vi "1-1.vi"() -> ()   [LabVIEW 2012]
doc: "© Copyright M. Ferrari 2000"
panel:
  out "LED":bool caption="Modificare le dimensioni e il colore del LED evidenziare il testo booleano. Provare, tramite l'opzione Show... a far apparire e scomparire tali informazioni"
  in  "?":dbl(knob)=12.0 min=12.0 max=35.0 scale=0.0..10.0 scale format="%.1f"
  out "Graph":dbl(graph) caption="Modificare i parametri del grafico: scale e colori"
  in  "?":bool
  in  "?":bool
  in  "Etichetta":dbl format="%.2f"
  in  "?":bool
  in  "?":bool
  in  "?":bool
  in  "?":bool
  in  "?":bool
  in  "?":bool
  # "ESERCIZIO 1-1"
  # "Assegnare un' etichetta\ne cancellare questa scritta"
  # "Riposizionare unitariamente\ni 4 interruttori"
  # "Creare un'etichetta libera e duplicarla,\nmodificando i font della copia"
  # "Modificare i limiti e provare a ruotare la manopola"
  # "Questa è un'etichetta libera, fare in modo\nche rimanga il testo senza cornice"
  # "Allineare orizzontalmente i 4 pulsanti ed equispaziarli."
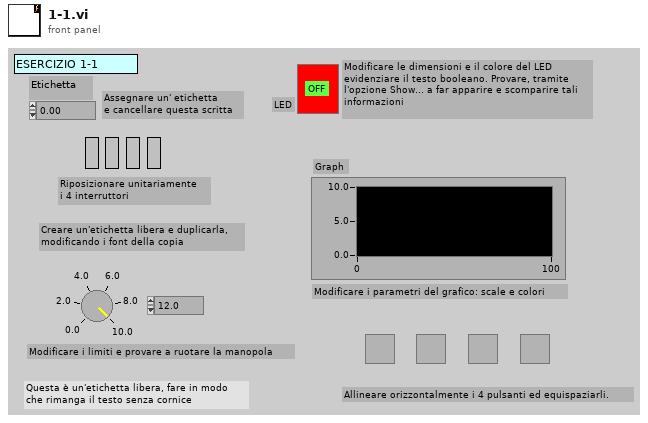
[diagram p1: front panel]
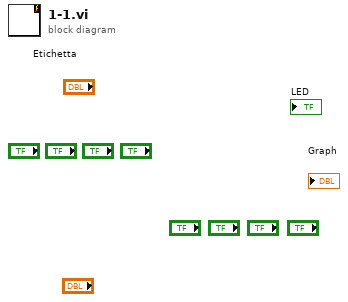
[diagram p0: block diagram]
diagram:
